vi "Register Channel.vi"(7 "Channel Array in":refnum<class "CIFChannels.lvclass">[](array[class]), 8 "error in (no error)":errorcluster, 9 "Channel":refnum<class "CIFChannels.lvclass">, 11 "CIFChannelMng in":refnum<class "CIFChannelMng.lvclass">) -> (0 "error out":errorcluster, 2 "Update Channel OOB":bool, 3 "CIFChannelMng out":refnum<class "CIFChannelMng.lvclass">, 5 "Channel Array out":refnum<class "CIFChannels.lvclass">[](array[class]))   [LabVIEW 2021, in "CIFChannelMng.lvclass"]
uses:
  CIFChannelMng.lvclass
  CIFChannelMng.lvclass/CIFChannelMng.ctl
  <vilib>/CIF Foundation/CIF Channels Core/ChannelCommon/ChannelCommon.lvlib
  <vilib>/CIF Foundation/CIF Channels Core/ChannelCommon/typedef/Errors.ctl
  <vilib>/CIF Foundation/CIF Channels Core/CIFChannels/CIFChannels.lvclass
  <vilib>/CIF Foundation/CIF Channels Core/CIFChannels/Typedef/Direction.ctl
  typedef/Channel List for OOB.ctl
  <vilib>/CIF Foundation/CIF Channels Core/CIFChannels/Typedef/Channel State.ctl
  <vilib>/CIF Foundation/CIF Channels Core/ChannelCommon/typedef/Channel Pattern.ctl
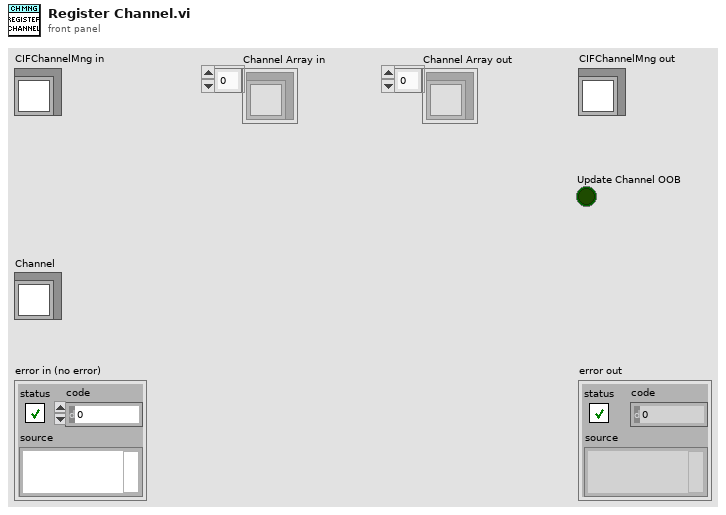
[diagram p1: front panel]
types:
  T1 = typedef "ChannelCommon.lvlib/Errors.ctl" = enum16{"gRPC Server Not Found", "Duplicate Channel", "Missing Channel", "Incorrect Type", "Flatten Error", "Unflatten Data", "Channel Length", "Plugin Connection", "gRPC Server Connection", "FIFO Unflatten", "Required Override", "Remove Not Found", "Not Supported"}
  T2 = typedef "CIFChannels.lvclass/Channel State.ctl" = enum16{"Creating", "Disconnected", "Connecting", "Connected", "Destroyed"}
  T3 = typedef "CIFChannelMng.lvclass/Channel List for OOB.ctl" = cluster{"Name":string, "Direction":T4, "Type":string, "Connected?":bool, "Connected Name":string, "Custom Config Data":u8[], "Forced?":bool, "Pattern":T5}
  T4 = typedef "CIFChannels.lvclass/Direction.ctl" = enum16{"Publisher", "Subscriber"}
  T5 = typedef "ChannelCommon.lvlib/Channel Pattern.ctl" = enum16{"Unknown", "Tag", "FIFO", "MultiFIFO"}
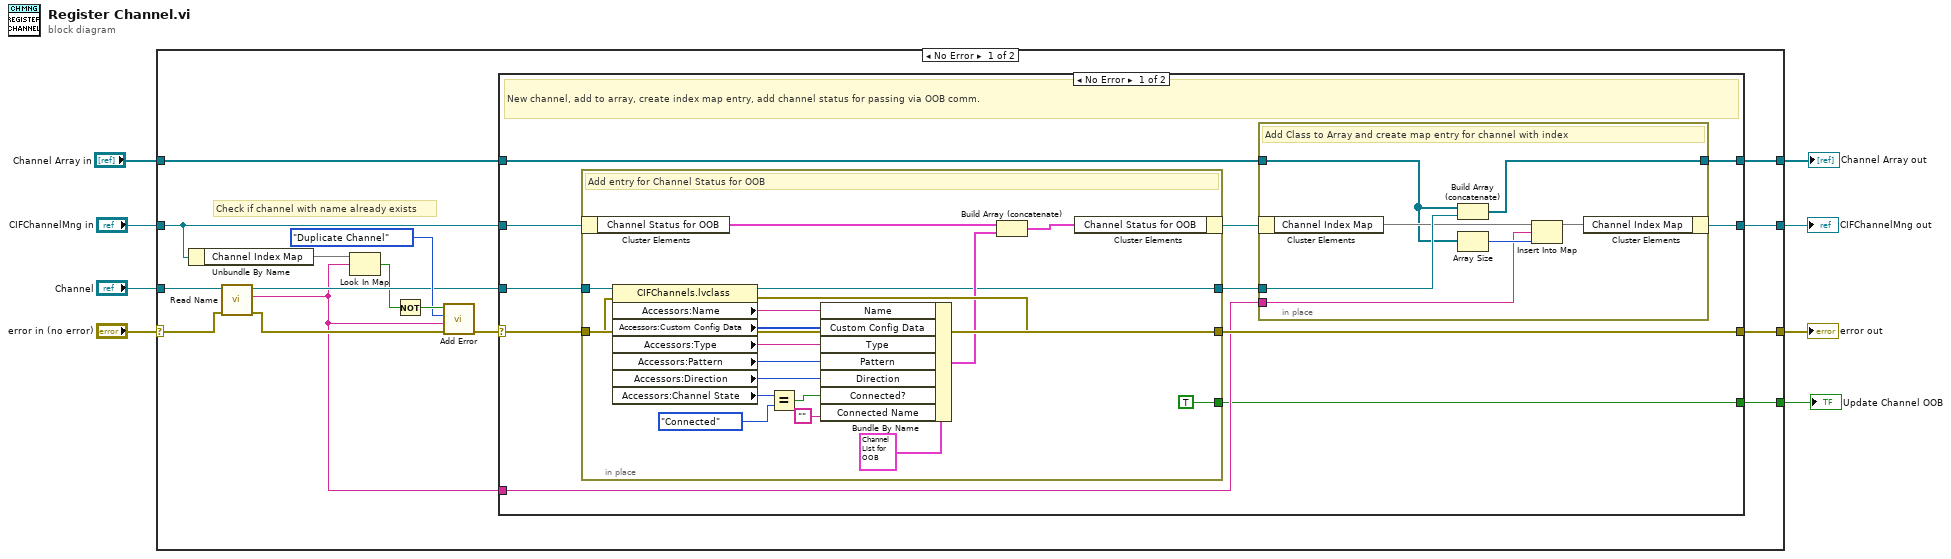
[diagram p0: block diagram]
diagram:
  n1 = case shown="No Error" "error in (no error)" {
    selector: "error in (no error)" -> [w20 w65]
    tunnel: [w19 w65] -> w7
    tunnel: [w17 w64] -> w5
    tunnel: "CIFChannelMng in" -> [w15 w64]
    tunnel: "Channel" -> [w21 _]
    tunnel: [w11 _] -> w3
    tunnel: "Channel Array in" -> [w10 w63]
    tunnel: [w9 w63] -> w1
    frame No Error {
      # "Check if channel with name already exists"
      n2 = Unbundle By Name(w15) -> ("Channel Index Map"=w14:map{string, i32})
      n3 = call <vilib>:"Read Name.vi"("error in (no error)"=w20, "CIFChannels in"=w21) -> ("error out"=w13:errorcluster, "Name"=w12:string, "CIFChannels out"=w18:refnum<class "CIFChannels.lvclass">)  [unwired: 7 in]
      n4 = Look In Map(map=w14, key=w12) -> (key not found?=w16:bool)  [unwired: 1 in, 1 out]
      n5 = Not(x=w16) -> (.not. x?=w23:bool)
      n6 = call <vilib>:"Add Error.vi"("error in (no error)"=w13, "String to Append"=w12, "Error"=Errors."Duplicate Channel", "Insert Error"=w23) -> ("error out"=w19:errorcluster)  [unwired: 7 in]
      n7 = case shown="No Error" w19 {
        selector: w19 -> [w27 w61]
        tunnel: w15 -> [w33 w62]
        tunnel: w18 -> [w28 _]
        tunnel: [w29 w62] -> w17
        tunnel: [w34 w61] -> _
        tunnel: w12 -> [w30 _]
        tunnel: [w26 _] -> w11
        tunnel: w10 -> [w25 w60]
        tunnel: [w24 w60] -> w9
        frame No Error {
          # "New channel, add to array, create index map entry, add channel status for passing via OOB comm."
          n8 = in-place {
            in-place-border: w28 -> [w59]
            in-place-border: w27 -> [w55]
            in-place-border: [w54] -> w34
            in-place-border: [w47] -> w31
            in-place-border: [TRUE ("Update OOB")] -> w26
            # "Add entry for Channel Status for OOB"
            n9 = in-place-cluster #1(w33) -> ("Channel Status for OOB"=w49:T3[])
            n10 = property class="CIFChannels.lvclass"(reference=w59, error in=w55) -> (reference out=w47:refnum<class "CIFChannels.lvclass">, error out=w54:errorcluster, "Accessors:Name"=w51:string, "Accessors:Custom Config Data"=w56:u8[], "Accessors:Type"=w57:string, "Accessors:Pattern"=w46:T5, "Accessors:Direction"=w52:T4, "Accessors:Channel State"=w44:T2)
            n11 = Equal?(x=w44, y=Channel_State."Connected") -> (x = y?=w45:bool)
            n12 = Bundle By Name(cluster=T3 {"Name"="", "Direction"=enum."Publisher", "Type"="", "Connected?"=FALSE, "Connected Name"="", "Custom Config Data"=[], "Forced?"=FALSE, "Pattern"=enum."Unknown"} ("Channel List"), "Name"=w51, "Custom Config Data"=w56, "Type"=w57, "Pattern"=w46, "Direction"=w52, "Connected?"=w45, "Connected Name"="") -> (w50:T3)
            n13 = Build Array (concatenate)(w49, w50) -> (w48:T3[])
            n14 = in-place-cluster #1("Channel Status for OOB"=w48) -> (w32:refnum<class "CIFChannelMng.lvclass">)
          }
          n15 = in-place {
            in-place-border: w31 -> [w41]
            in-place-border: w30 -> [w37]
            in-place-border: w25 -> [w36]
            in-place-border: [w35] -> w24
            # "Add Class to Array and create map entry for channel with index"
            n16 = in-place-cluster #2(w32) -> ("Channel Index Map"=w40:map{string, i32})
            n17 = Build Array (concatenate)(w36, w41) -> (w35:refnum<class "CIFChannels.lvclass">[])
            n18 = Array Size(array=w36) -> (size(s)=w38:i32)
            n19 = Insert Into Map(map in=w40, key=w37, value=w38) -> (map out=w39:map{string, i32})  [unwired: 2 out]
            n20 = in-place-cluster #2("Channel Index Map"=w39) -> (w29:refnum<class "CIFChannelMng.lvclass">)
          }
        }
        frame Error {
        }
      }
    }
    frame Error {
    }
  }
  "error out" <- w7
  "CIFChannelMng out" <- w5
  "Update Channel OOB" <- w3
  "Channel Array out" <- w1
